vi "2086查询单参数.vi"(8 "error in (no error)":errorcluster, 9 "索引":i32, 10 "table":string, 11 "database":string="database1.mdb") -> (0 "error out":errorcluster, 1 "拆分数据":bool, 2 "database溢出":bool, 3 "data":string[][](array[string]), 5 "有数据":bool)   [LabVIEW 2016, in "数据传输系统-02.lvlib"]
uses:
  <vilib>/Utility/sysdir.llb/System Directory Type.ctl
  <vilib>/addons/database/Connection.llb/DB Tools Open Connec (String).vi
  <vilib>/addons/database/Connection.llb/Conn Execute.vi
  <vilib>/addons/database/Recordset.llb/Rec Fetch Recordset Data (R).vi
  <vilib>/addons/database/Recordset.llb/Rec Destroy - Connection.vi
  <vilib>/addons/database/_DB Variant To Data/Database Variant To Data.xnode
  <vilib>/addons/database/NI_Database_API.lvlib
panel:
  out "连接的字符串":string
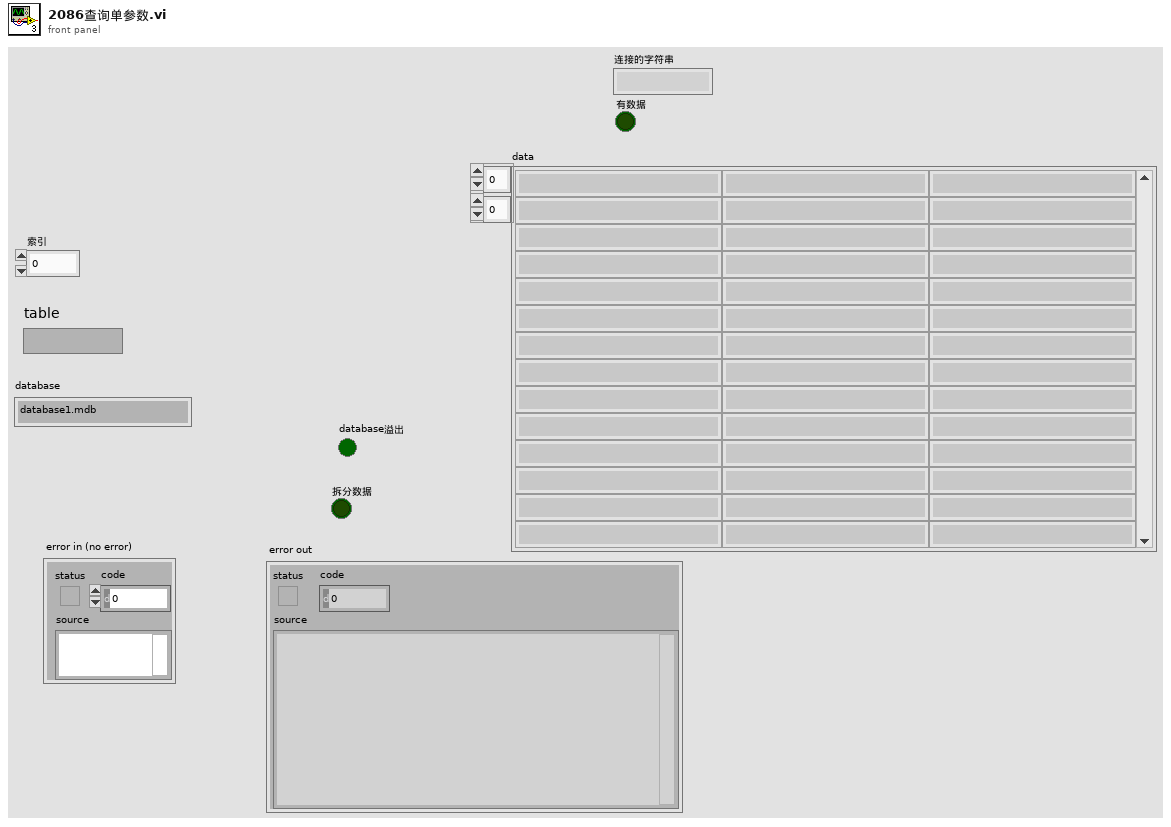
[diagram p1: front panel]
types:
  T1 = typedef "System Directory Type.ctl" = i32
  T2 = cluster{"time1":string, "time2":string, "time3":string, "time4":string, "time5":string, "time6":string, "time7":string, "time8":string, "time9":string, "time10":string, "time11":string, "time12":string, "time13":string, "time14":string, "time15":string, "time16":string, "time17":string, "time18":string, "time19":string, "time20":string, "time21":string, "time22":string, "time23":string, "time24":string, "time25":string, "time26":string, "time27":string, "time28":string, "time29":string, "time30":string, "time31":string, "time32":string, "time33":string, "time34":string, "time35":string, "time36":string, "time37":string, "time38":string, "time39":string, "time40":string, "time41":string, "time42":string, "time43":string, "time44":string, "time45":string, "time46":string, "time47":string, "time48":string, "time49":string, "time50":string, "time51":string, "time52":string, "time53":string, "time54":string, "time55":string, "time56":string, "time57":string, "time58":string, "time59":string, "time60":string, "time61":string, "time62":string, "time63":string, "time64":string, "time65":string, "time66":string, "time67":string, "time68":string, "time69":string, "time70":string, "time71":string, "time72":string, "time73":string, "time74":string, "time75":string, "time76":string}
  T3 = typedef "NI_Database_API.lvlib/Conn ObjectReference.ctl" = refnum<k1>
  T4 = typedef "NI_Database_API.lvlib/Rec ObjectReference.ctl" = refnum<k1>
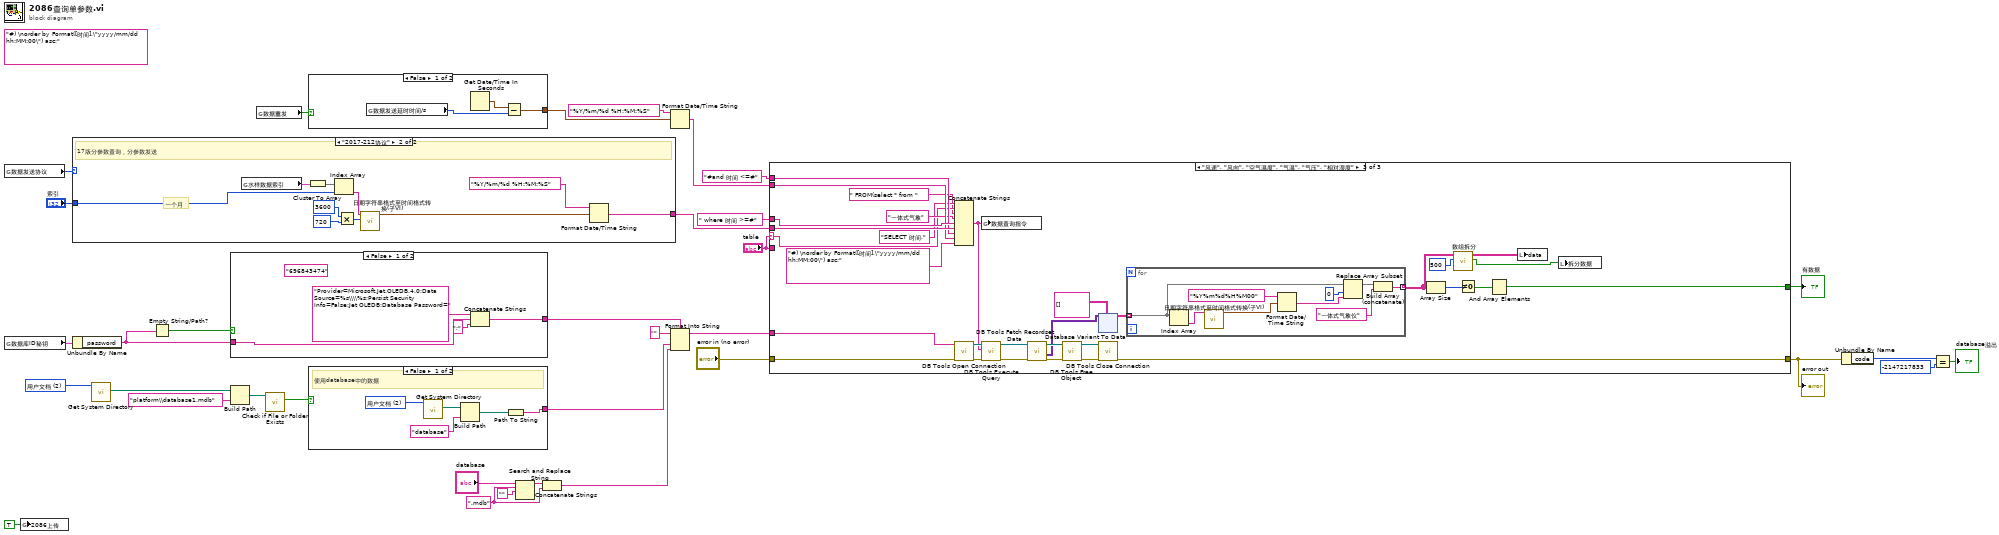
[diagram p0: block diagram]
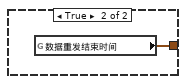
[diagram p2: hidden frame]
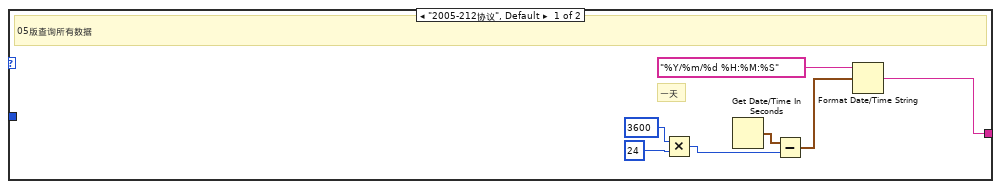
[diagram p3: hidden frame]
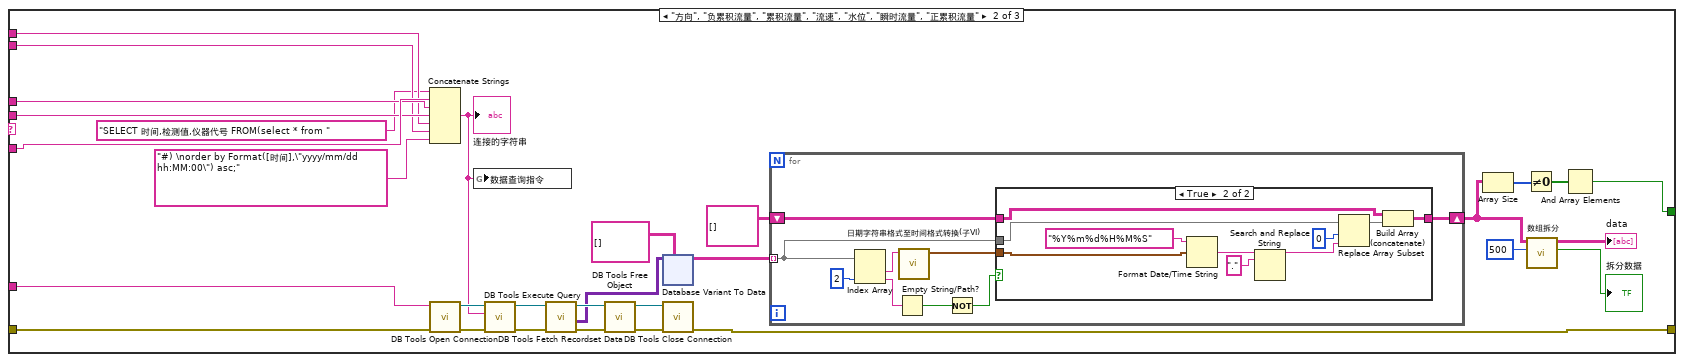
[diagram p5: hidden frame]
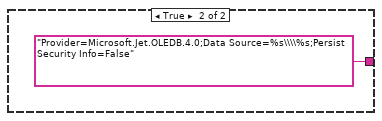
[diagram p7: hidden frame]
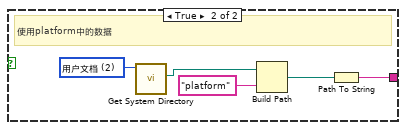
[diagram p8: hidden frame]
diagram:
  (unwired) "#) \norder by Format([时间],\"yyyy/mm/dd hh:MM:00\") asc;" ("字符串")
  w19 = ".mdb" ("搜索字符串")
  w29 = T1 2 items=["用户目录"=0, "用户桌面"=1, "用户文档"=2, "用户应用程序数据"=3, "用户设置"=4, "用户临时目录"=5, "公共文档"=6, "公共应用程序数据"=7, "公共设置"=8, "公共缓存"=13, "系统核心库"=9, "系统安装库"=10, "应用程序文件"=11, "启动盘根目录"=12] ("system directory type")
  n1 = global read "断电保存全局.vi" "数据发送协议"() -> (w10:enum16{"2005-212协议", "2017-212协议"})
  n2 = global read "外部交互全局.vi" "数据库ID秘钥"() -> (w22:cluster{"userID":string, "password":string})
  n3 = global write "全局1.vi" "2086上传"(TRUE ("2086上传")) -> ()
  n4 = case shown="\"2017-212协议\"" w10 {
    tunnel: [w40 w43] -> w12
    tunnel: "索引" -> [_ w49]
    frame "2005-212协议", Default {
      # "一天"
      # "05版查询所有数据"
      n5 = Multiply(x=3600, y=24) -> (x*y=w35:i32)
      n6 = Get Date/Time In Seconds() -> (seconds since 1Jan1904=w39:timestamp)
      n7 = Subtract(x=w39, y=w35) -> (x-y=w38:timestamp)
      n8 = Format Date/Time String(time format string (%c)="%Y/%m/%d %H:%M:%S" ("时间格式字符串(%c)"), seconds (now)=w38) -> (date/time string=w40:string)  [unwired: 1 in]
    }
    frame "2017-212协议" {
      # "一个月"
      # "17版分参数查询，分参数发送"
      n9 = global read "全局 水样时间.vi" "水样数据索引"() -> (w50:T2)
      n10 = Cluster To Array(cluster=w50) -> (array=w51:string[])
      n11 = Index Array(array=w51, index=w49) -> (element=w48:string)
      n12 = Multiply(x=3600, y=720) -> (x*y=w45:i32)
      n13 = call "日期字符串格式至时间格式转换(子VI).vi"("数值"=w45, "data[0]"=w48) -> ("time stamp"=w42:timestamp)  [unwired: 9 in]
      n14 = Format Date/Time String(time format string (%c)="%Y/%m/%d %H:%M:%S" ("时间格式字符串(%c)"), seconds (now)=w42) -> (date/time string=w43:string)  [unwired: 1 in]
    }
  }
  n15 = Unbundle By Name(w22) -> ("password"=w24:string)
  n16 = call <vilib>:"Get System Directory.vi"("system directory type"=w29) -> ("system directory"=w30:path)  [unwired: 10 in]
  n17 = Empty String/Path?(string/path=w24) -> (empty?=w2:bool)
  n18 = case shown="False" w2 {
    tunnel: [w53 "Provider=Microsoft.Jet.OLEDB.4.0;Data Source=%s\\\\%s;Persist Security Info=False" ("格式字符串")] -> w23
    tunnel: w24 -> [w52 _]
    frame False {
      (unwired) "696843474" ("格式字符串")
      n19 = Concatenate Strings("Provider=Microsoft.Jet.OLEDB.4.0;Data Source=%s\\\\%s;Persist Security Info=False;Jet OLEDB:Database Password=" ("格式字符串"), w52, ";" ("字符串")) -> (w53:string)
    }
    frame True {
    }
  }
  n20 = Build Path(base path=w30, name or relative path="platform\\database1.mdb" ("condition")) -> (appended path=w28:path)
  n21 = global read "断电保存全局.vi" "数据重发"() -> (w9:bool)
  n22 = call <vilib>:"Check if File or Folder Exists.vi"("path"=w28) -> ("file or folder exists?"=w26:bool)  [unwired: 8 in, 2 out]
  n23 = case shown="False" w9 {
    tunnel: [w57 w60] -> w7
    frame False {
      n24 = global read "断电保存全局.vi" "数据发送延时时间/s"() -> (w58:i32)
      n25 = Get Date/Time In Seconds() -> (seconds since 1Jan1904=w59:timestamp)
      n26 = Subtract(x=w59, y=w58) -> (x-y=w57:timestamp)
    }
    frame True {
      n27 = global read "断电保存全局.vi" "数据重发结束时间"() -> (w60:timestamp)
    }
  }
  n28 = case shown="False" w26 {
    tunnel: [w61 w66] -> w25
    frame False {
      w64 = T1 2 items=["用户目录"=0, "用户桌面"=1, "用户文档"=2, "用户应用程序数据"=3, "用户设置"=4, "用户临时目录"=5, "公共文档"=6, "公共应用程序数据"=7, "公共设置"=8, "公共缓存"=13, "系统核心库"=9, "系统安装库"=10, "应用程序文件"=11, "启动盘根目录"=12] ("system directory type")
      # "使用database中的数据"
      n29 = call <vilib>:"Get System Directory.vi"("system directory type"=w64) -> ("system directory"=w63:path)  [unwired: 10 in]
      n30 = Build Path(base path=w63, name or relative path="database" ("condition")) -> (appended path=w65:path)
      n31 = Path To String(path=w65) -> (string=w61:string)
    }
    frame True {
      w70 = T1 2 items=["用户目录"=0, "用户桌面"=1, "用户文档"=2, "用户应用程序数据"=3, "用户设置"=4, "用户临时目录"=5, "公共文档"=6, "公共应用程序数据"=7, "公共设置"=8, "公共缓存"=13, "系统核心库"=9, "系统安装库"=10, "应用程序文件"=11, "启动盘根目录"=12] ("system directory type")
      # "使用platform中的数据"
      n32 = call <vilib>:"Get System Directory.vi"("system directory type"=w70) -> ("system directory"=w69:path)  [unwired: 10 in]
      n33 = Build Path(base path=w69, name or relative path="platform" ("condition")) -> (appended path=w67:path)
      n34 = Path To String(path=w67) -> (string=w66:string)
    }
  }
  n35 = Search and Replace String(input string="database", search string=w19, replace string="") -> (result string=w20:string)  [unwired: 5 in, 3 out]
  n36 = Concatenate Strings(w20, w19) -> (w17:string)
  n37 = Format Date/Time String(time format string (%c)="%Y/%m/%d %H:%M:%S" ("时间格式字符串(%c)"), seconds (now)=w7) -> (date/time string=w6:string)  [unwired: 1 in]
  n38 = Format Into String(format string=w23, initial string="" ("初始字符串"), w25, w17) -> (resulting string=w13:string)  [unwired: 1 in, 1 out]
  n39 = case shown="\"风速\", \"风向\", \"空气温度\", \"气温\", \"气压\", \"相对湿度\"" "table" {
    selector: "table" -> [_ _ w169]
    tunnel: "table" -> [_ w97 _]
    tunnel: " where 时间 >=#" -> [_ w96 w191]
    tunnel: w12 -> [_ w95 w190]
    tunnel: "#and 时间 <=#" -> [_ w94 w189]
    tunnel: w6 -> [_ w93 w188]
    tunnel: "error in (no error)" -> [w71 w84 w180]
    tunnel: [w71 w87 w183] -> w14
    tunnel: w13 -> [_ w86 w182]
    tunnel: [_ w72 w172] -> w1
    frame "假", Default {
    }
    frame "方向", "负累积流量", "累积流量", "流速", "水位", "瞬时流量", "正累积流量" {
      n40 = Concatenate Strings("SELECT 时间,检测值,仪器代号 FROM(select * from " ("连接的字符串"), w97, w96, w95, w94, w93, "#) \norder by Format([时间],\"yyyy/mm/dd hh:MM:00\") asc;" ("字符串")) -> (w76:string)
      "连接的字符串" <- w76
      n41 = call-poly <vilib>:"DB Tools Open Connection.vi"("error in (no error)"=w84, "connection information"=w86) -> ("error out"=w83:errorcluster, "connection reference"=w85:T3)  [unwired: 6 in]
      n42 = global write "全局 水样时间.vi" "数据查询指令"(w76) -> ()
      n43 = call-poly <vilib>:"DB Tools Execute Query.vi"("error in (no error)"=w83, "SQL query"=w76, "connection reference"=w85) -> ("error out"=w101:errorcluster, "recordset reference"=w99:T4)  [unwired: 5 in]
      n44 = call-poly <vilib>:"DB Tools Fetch Recordset Data.vi"("error in (no error)"=w101, "recordset reference"=w99) -> ("error out"=w98:errorcluster, "recordset data"=w92:variant[][], "recordset reference out"=w100:T4)  [unwired: 3 in]
      n45 = call-poly <vilib>:"DB Tools Free Object.vi"("error in (no error)"=w98, "recordset reference"=w100) -> ("error out"=w88:errorcluster, "connection reference"=w89:T3)  [unwired: 8 in]
      n46 = xnode "Database Variant To Data"("database variant"=w92, "type"=string[][] []) -> ("data"=w81:string[][])  [unwired: 1 in, 1 out]
      n47 = call <vilib>:"DB Tools Close Connection.vi"("error in (no error)"=w88, "connection reference"=w89) -> ("error out"=w87:errorcluster)  [unwired: 5 in]
      n48 = for {
        tunnel: w81 -> [w108] mode=indexing
        shift-right: [w103] -> w75
        shift-left: string[][] [] -> [w110]
        n49 = Index Array(array=w108, index #2=2 ("索引")) -> (element #1=w109:string, element #2=w105:string)  [unwired: 1 in]
        n50 = Empty String/Path?(string/path=w105) -> (empty?=w104:bool)
        n51 = call "日期字符串格式至时间格式转换(子VI).vi"("data[0]"=w109) -> ("time stamp"=w107:timestamp)  [unwired: 10 in]
        n52 = Not(x=w104) -> (.not. x?=w102:bool)
        n53 = case shown="True" w102 {
          tunnel: w108 -> [_ w118]
          tunnel: [_ w119] -> w103
          tunnel: w110 -> [_ w120]
          tunnel: w107 -> [_ w115]
          frame False {
          }
          frame True {
            n54 = Format Date/Time String(time format string (%c)="%Y%m%d%H%M%S" ("时间格式字符串(%c)"), seconds (now)=w115) -> (date/time string=w113:string)  [unwired: 1 in]
            n55 = Search and Replace String(input string=w113, search string="." ("搜索字符串")) -> (result string=w114:string)  [unwired: 6 in, 3 out]
            n56 = Replace Array Subset(array=w118, new element=w114, index=0 ("索引")) -> (w111:string[])
            n57 = Build Array (concatenate)(w120, w111) -> (w119:string[][])
          }
        }
      }
      n58 = Array Size(array=w75) -> (size(s)=w74:i32[])
      n59 = Not Equal To 0?(x=w74) -> (x != 0?=w73:bool[])
      n60 = call "数组拆分.vi"("拆分大小"=500, "输入数据"=w75) -> ("拆分数据"=→"拆分数据":bool, "输出数组"=→"data":string[][])  [unwired: 8 in]
      n61 = And Array Elements(Boolean array=w73) -> (logical AND=w72:bool)
    }
    frame "风速", "风向", "空气温度", "气温", "气压", "相对湿度" {
      n62 = Concatenate Strings("SELECT 时间," ("连接的字符串"), w169, " FROM(select * from " ("连接的字符串"), "一体式气象" ("字符串"), w191, w190, w189, w188, "#) \norder by Format([时间],\"yyyy/mm/dd hh:MM:00\") asc;" ("字符串")) -> (w175:string)
      n63 = call-poly <vilib>:"DB Tools Open Connection.vi"("error in (no error)"=w180, "connection information"=w182) -> ("error out"=w179:errorcluster, "connection reference"=w181:T3)  [unwired: 6 in]
      n64 = global write "全局 水样时间.vi" "数据查询指令"(w175) -> ()
      n65 = call-poly <vilib>:"DB Tools Execute Query.vi"("error in (no error)"=w179, "SQL query"=w175, "connection reference"=w181) -> ("error out"=w195:errorcluster, "recordset reference"=w193:T4)  [unwired: 5 in]
      n66 = call-poly <vilib>:"DB Tools Fetch Recordset Data.vi"("error in (no error)"=w195, "recordset reference"=w193) -> ("error out"=w192:errorcluster, "recordset data"=w187:variant[][], "recordset reference out"=w194:T4)  [unwired: 3 in]
      n67 = call-poly <vilib>:"DB Tools Free Object.vi"("error in (no error)"=w192, "recordset reference"=w194) -> ("error out"=w184:errorcluster, "connection reference"=w185:T3)  [unwired: 8 in]
      n68 = xnode "Database Variant To Data"("database variant"=w187, "type"=string[][] []) -> ("data"=w178:string[][])  [unwired: 1 in, 1 out]
      n69 = call <vilib>:"DB Tools Close Connection.vi"("error in (no error)"=w184, "connection reference"=w185) -> ("error out"=w183:errorcluster)  [unwired: 5 in]
      n70 = for {
        tunnel: w178 -> [w199] mode=indexing
        tunnel: [w203] -> w166 mode=indexing
        n71 = Index Array(array=w199) -> (element=w200:string)  [unwired: 1 in]
        n72 = call "日期字符串格式至时间格式转换(子VI).vi"("data[0]"=w200) -> ("time stamp"=w201:timestamp)  [unwired: 10 in]
        n73 = Format Date/Time String(time format string (%c)="%Y%m%d%H%M00" ("时间格式字符串(%c)"), seconds (now)=w201) -> (date/time string=w198:string)  [unwired: 1 in]
        n74 = Replace Array Subset(array=w199, new element=w198, index=0 ("索引")) -> (w197:string[])
        n75 = Build Array (concatenate)(w197, "一体式气象仪" ("字符串")) -> (w203:string[])
      }
      n76 = Array Size(array=w166) -> (size(s)=w174:i32[])
      n77 = call "数组拆分.vi"("拆分大小"=500, "输入数据"=w166) -> ("拆分数据"=w167:bool, "输出数组"=w168:string[][])  [unwired: 8 in]
      n78 = Not Equal To 0?(x=w174) -> (x != 0?=w173:bool[])
      n79 = And Array Elements(Boolean array=w173) -> (logical AND=w172:bool)
      n80 = local write "data"(w168) -> ()
      n81 = local write "拆分数据"(w167) -> ()
    }
  }
  "error out" <- w14
  "有数据" <- w1
  n82 = Unbundle By Name(w14) -> ("code"=w34:i32)
  n83 = Equal?(x=w34, y=-2147217833 ("code")) -> (x = y?=→"database溢出":bool)
